vi "Continue Start.vi"(8 "Error in":errorcluster, 11 "Com in":refnum<visa-resource-name>) -> (0 "error out":errorcluster caption="Error out", 3 "Com out":refnum<visa-resource-name>)   [LabVIEW 2020]
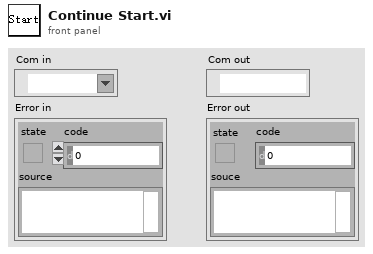
[diagram p1: front panel]
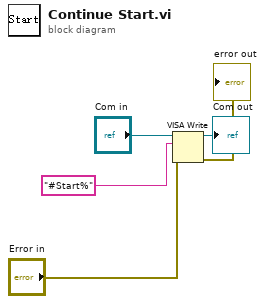
[diagram p0: block diagram]
diagram:
  n1 = VISA Write(VISA resource name="Com in", write buffer="#Start%" ("字符串"), error in (no error)="Error in") -> (VISA resource name out=→"Com out":refnum<visa-resource-name>, error out=→"error out":errorcluster)  [unwired: 1 out]
